vi "discrete signal.vi"() -> ()   [LabVIEW 2017]
panel:
  out "main signal":waveform(dbl)[](graph)
  out "discrete signal":waveform(dbl)(graph)
  out "discrete signal":waveform(dbl)
  in  "path 3":path
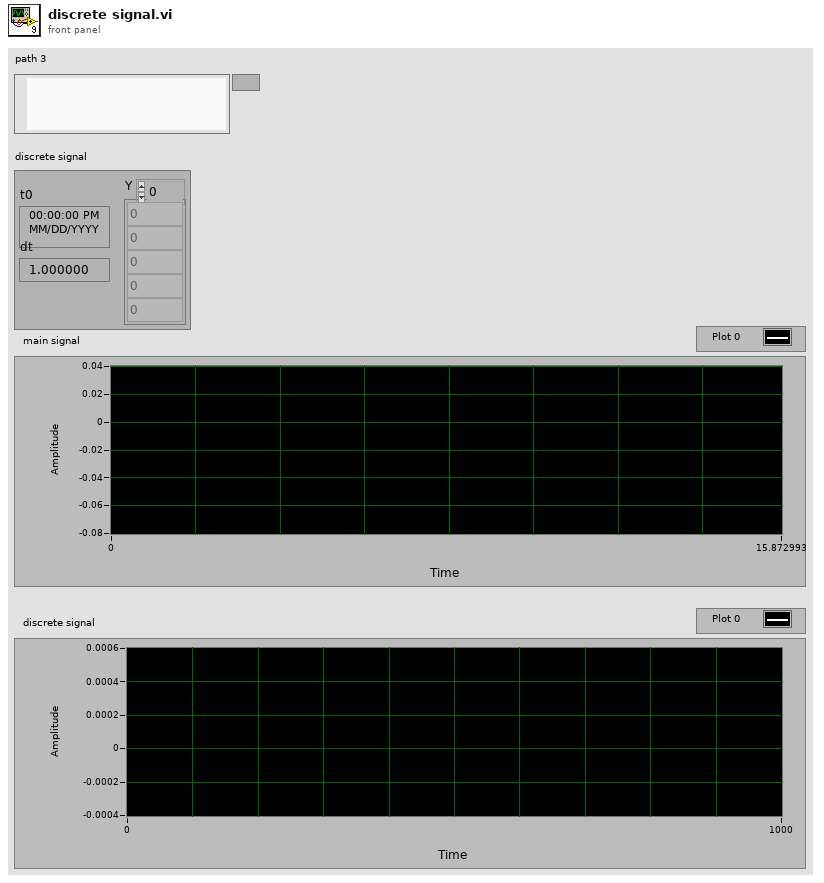
[diagram p1: front panel]
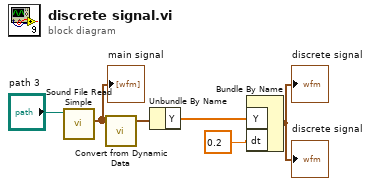
[diagram p0: block diagram]
diagram:
  n1 = call <vilib>:"Sound File Read Simple.vi"("path"="path 3") -> ("data"=w3:waveform(dbl)[])  [unwired: 7 in, 3 out]
  "main signal" <- w3
  n2 = call "Convert from Dynamic Data"("Dynamic Data Type"=w3) -> ("Waveform"=w2:waveform(dbl))  [unwired: 3 in]
  n3 = Unbundle By Name(w2) -> ("Y"=w1:dbl[])
  n4 = Bundle By Name("Y"=w1, "dt"=0.2) -> (→"discrete signal" →"discrete signal":waveform(dbl))  [unwired: 1 in]
